vi "client.vi"(0 "设备信息":T1={"设备名称"="", "操作人员"="", "设备状态"=enum."设备正常", "附加信息"=""}) -> ()   [LabVIEW 2019]
uses:
  Global_Variable/Global.vi
panel:
  in  "服务器关闭":string="服务器VI关闭了连接。"
  in  "停止":bool
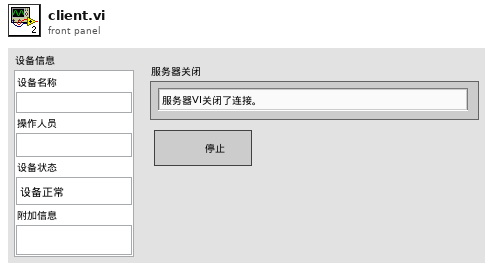
[diagram p1: front panel]
types:
  T1 = cluster{"设备名称":string, "操作人员":string, "设备状态":enum16{"设备离线", "设备正常", "设备缺料", "设备故障", "质量报警"}, "附加信息":string}
  T2 = cluster{"设备名称":bool, "操作人员":bool, "设备状态":bool, "附加信息":bool}
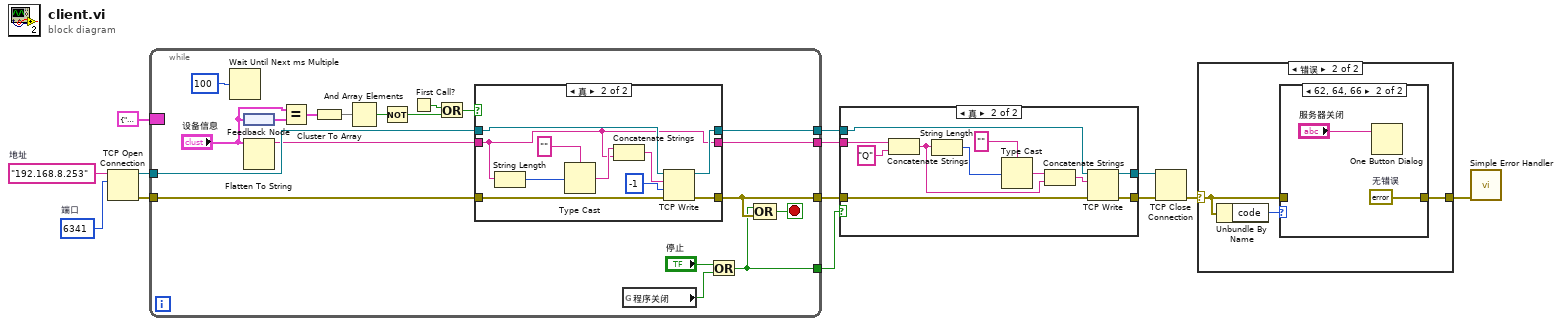
[diagram p0: block diagram]
diagram:
  w12 = u16 6341  # 端口
  w13 = "192.168.8.253"  # 地址
  n1 = TCP Open Connection(address=w13, remote port or service name=w12) -> (connection ID=w11:refnum<k5>, error out=w10:errorcluster)  [unwired: 1 in, 2 out]
  n2 = while {
    tunnel: [w15] -> w5
    tunnel: [w30] -> w9
    tunnel: [w27] -> w7
    tunnel: w10 -> [w31]
    tunnel: w11 -> [w32]
    tunnel: [w20] -> w2
    border: T1 {"设备名称"="", "操作人员"="", "设备状态"=enum."设备正常", "附加信息"=""} ("设备信息") -> [_]
    stop <- w29 stop-if-true
    n3 = Wait Until Next ms Multiple(millisecond multiple=u32 100 ("毫秒倍数")) -> ()  [unwired: 1 out]
    n4 = feedback-in #1("设备信息") -> ()
    n5 = feedback #1() -> (w24:T1)
    n6 = Flatten To String(anything="设备信息") -> (data string=w21:string)  [unwired: 3 in, 2 out]
    n7 = Equal?(x="设备信息", y=w24) -> (x = y?=w23:T2)
    n8 = Cluster To Array(cluster=w23) -> (array=w22:bool[])
    n9 = And Array Elements(Boolean array=w22) -> (logical AND=w19:bool)
    n10 = Not(x=w19) -> (.not. x?=w16:bool)
    n11 = First Call?() -> (First Call?: T/F=w17:bool)
    n12 = Or(x=w17, y=w16) -> (x .or. y?=w18:bool)
    n13 = case shown="真" w18 {
      tunnel: w32 -> [w35 w45]
      tunnel: w31 -> [w34 w44]
      tunnel: [w35 w43] -> w30
      tunnel: [w34 w42] -> w27
      tunnel: w21 -> [w33 w36]
      tunnel: [w33 w36] -> w20
      frame False {
      }
      frame True {
        n14 = String Length(string=w36) -> (length=w40:i32)
        n15 = Type Cast(type="", x=w40) -> (*(type *) &x=w38:string)
        n16 = Concatenate Strings(w38, w36) -> (w37:string)
        n17 = TCP Write(connection ID=w45, data in=w37, error in (no error)=w44, 9:-1) -> (connection ID out=w43:refnum<k5>, error out=w42:errorcluster)  [unwired: 1 out]
      }
    }
    n18 = global read "Global.vi" "程序关闭"() -> (w14:bool)
    n19 = Or(x="停止", y=w14) -> (x .or. y?=w15:bool)
    n20 = Compound Arithmetic op=OR ("复合运算")(w15, w27) -> (w29:bool)
  }
  n21 = case shown="真" w5 {
    tunnel: w9 -> [w47 w58]
    tunnel: [w47 w56] -> w8
    tunnel: w7 -> [w46 w57]
    tunnel: [w46 w55] -> w6
    tunnel: w2 -> [_ w53]
    frame False {
    }
    frame True {
      n22 = Concatenate Strings(w53, "Q") -> (w49:string)
      n23 = String Length(string=w49) -> (length=w52:i32)
      n24 = Type Cast(type="", x=w52) -> (*(type *) &x=w50:string)
      n25 = Concatenate Strings(w50, w49) -> (w48:string)
      n26 = TCP Write(connection ID=w58, data in=w48, error in (no error)=w57) -> (connection ID out=w56:refnum<k5>, error out=w55:errorcluster)  [unwired: 2 out]
    }
  }
  n27 = TCP Close Connection(connection ID=w8, error in (no error)=w6) -> (error out=w4:errorcluster)  [unwired: 2 out]
  n28 = case shown="错误" w4 {
    selector: w4 -> [w59 w61]
    tunnel: [w59 w60] -> w3
    frame No Error {
    }
    frame Error {
      n29 = Unbundle By Name(w61) -> ("code"=w62:i32)
      n30 = case shown="62, 64, 66" w62 {
        tunnel: w61 -> [w63 _]
        tunnel: [w63 w65] -> w60
        frame Default {
        }
        frame 62, 64, 66 {
          w65 = errorcluster {"status"=FALSE, "code"=0, "source"=""}  # 无错误
          n31 = One Button Dialog(message="服务器关闭") -> ()  [unwired: 1 in, 1 out]
        }
      }
    }
  }
  n32 = call <vilib>:"Simple Error Handler.vi"("error in (no error)"=w3) -> ()  [unwired: 1 in, 8 out]
